vi "Actor Core.vi"(8 "error in":errorcluster, 11 "Tools View in":refnum<class "Tools View.lvclass">) -> (0 "error out":errorcluster, 3 "Actor out":refnum<class "Actor.lvclass">)   [LabVIEW 2020, in "Tools View.lvlib" / "Tools View.lvclass"]
doc: "(<B>Filename</B>: Actor Framework.lvlib:Actor.lvclass:Actor Core.vi)\n\nReceives messages to the actor, reacts to them, and initiates any error handling that may shut the actor down.\n\nDescendant classes may override this VI to append parallel tasks for the actor to complete while it handles messages. Overrides use the Call Parent Method node."
uses:
  Tools View.lvclass
  C:/Program Files/National Instruments/LabVIEW 2020/vi.lib/ActorFramework/Actor/Actor.lvclass
  <vilib>/ActorFramework/Actor/Actor.lvclass
  Tools View.lvclass/Tools View.ctl
  <vilib>/ActorFramework/Actor/Actor.lvclass/Actor.ctl
  <vilib>/ActorFramework/Message Enqueuer/Message Enqueuer.lvclass/Message Enqueuer.ctl
  Type Definitions/Tool Buttons.ctl
  Tools View Messages/Broadcast Tool Buttons Pressed Msg/Broadcast Tool Buttons Pressed Msg.lvclass/Broadcast Tool Buttons Pressed Msg.ctl
  <vilib>/ActorFramework/Message Enqueuer/Init from Existing Queue.vi
  <vilib>/ActorFramework/Message Enqueuer/Enqueue.vi
  Tools View Messages/Broadcast Tool Buttons Pressed Msg/Broadcast Tool Buttons Pressed Msg.lvclass
  C:/Program Files/National Instruments/LabVIEW 2020/vi.lib/ActorFramework/Message/Message.lvclass
  <vilib>/ActorFramework/Message Priority Queue/Priority Enqueue.vi
  <vilib>/ActorFrameworkMVC/Abstract View/Abstract View/Abstract View.lvclass
  <vilib>/ActorFramework/Message Enqueuer/Message Enqueuer.lvclass
panel:
  in  "Disabled Crop Button":bool
  in  "Disabled Deselect Button":bool
  in  "Tool Buttons":T1(radio)
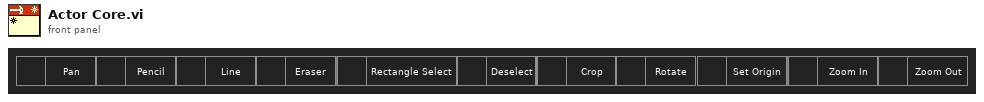
[diagram p1: front panel]
types:
  T1 = enum32{"Pan Button", "Pencil Button", "Line Button", "Eraser Button", "Rectangle Select Button", "Deselect Button", "Crop Button", "Rotate Button", "Set Origin Button", "Zoom In Button", "Zoom Out Button"}
  T2 = enum8{"Enabled", "Disabled", "Disabled and Grayed Out"}
  T3 = typedef "Tool Buttons.ctl" = enum32{"Pan Button", "Pencil Button", "Line Button", "Eraser Button", "Rectangle Select Button", "Deselect Button", "Crop Button", "Rotate Button", "Set Origin Button", "Zoom In Button", "Zoom Out Button"}
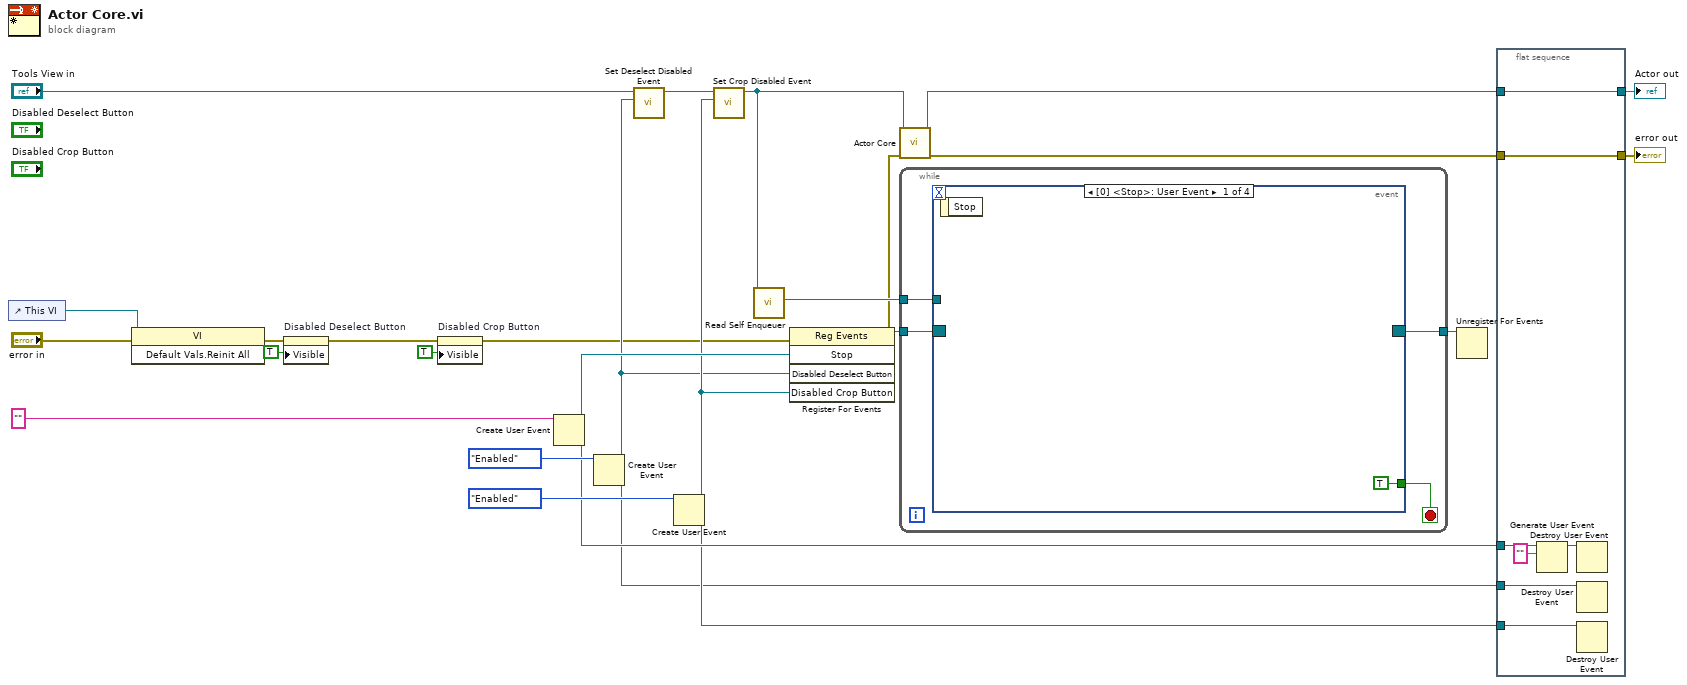
[diagram p0: block diagram]
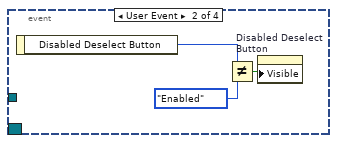
[diagram p2: hidden frame]
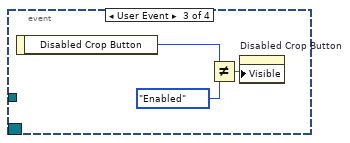
[diagram p3: hidden frame]
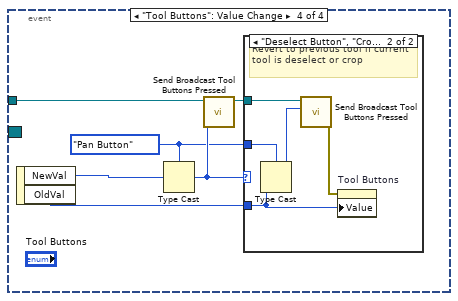
[diagram p4: hidden frame]
diagram:
  n1 = control-ref of="This VI"() -> (w6:refnum<vi>)
  n2 = invoke class="VI" method="Default Vals.Reinit All"(reference=w6, error in="error in") -> (error out=w5:errorcluster)  [unwired: 1 in, 2 out]
  n3 = property on="Disabled Deselect Button" class="Bool"(error in=w5, "Visible"=TRUE) -> (error out=w4:errorcluster)  [unwired: 1 in, 1 out]
  n4 = property on="Disabled Crop Button" class="Bool"(error in=w4, "Visible"=TRUE) -> (error out=w3:errorcluster)  [unwired: 1 in, 1 out]
  n5 = Create User Event(user event datatype="" ("Stop")) -> (user event=w18:refnum<user-event>)  [unwired: 1 in, 1 out]
  n6 = Create User Event(user event datatype=T2."Enabled" ("Disabled Deselect Button")) -> (user event=w9:refnum<user-event>)  [unwired: 1 in, 1 out]
  n7 = call "Set Deselect Disabled Event.vi"("Deselect Disabled Event"=w9, "Tools View in"="Tools View in") -> ("Tools View out"=w11:refnum<class "Tools View.lvclass">)  [unwired: 9 in]
  n8 = Create User Event(user event datatype=T2."Enabled" ("Disabled Crop Button")) -> (user event=w10:refnum<user-event>)  [unwired: 1 in, 1 out]
  n9 = call "Set Crop Disabled Event.vi"("Crop Disabled Event"=w10, "Tools View in"=w11) -> ("Tools View out"=w7:refnum<class "Tools View.lvclass">)  [unwired: 9 in]
  n10 = call <vilib>:"Read Self Enqueuer.vi"("Actor"=w7) -> ("Self Enqueuer"=w19:refnum<class "Message Enqueuer.lvclass">)  [unwired: 10 in]
  n11 = register-events(error in=w3, w18, w9, w10) -> (reference out=w20:refnum<event-registration>, error out=w12:errorcluster)  [unwired: 1 in]
  n12 = call-parent "Actor Core.vi"("error in"=w12, "Abstract View in"=w7) -> ("error out"=w15:errorcluster, "Actor out"=w14:refnum<class "Actor.lvclass">)  [unwired: 8 in]
  n13 = while {
    tunnel: w20 -> [w28]
    tunnel: [w27] -> w21
    tunnel: w19 -> [w25]
    stop <- w26 stop-if-true
    n14 = event shown="[0] <Stop>: User Event" {
      selector: w28 -> [_ _ _ _]
      dyn-events: [_ _ _ _] -> w27
      timeout: _ -> [_ _ _ _]
      tunnel: [TRUE _ _ _] -> w26
      tunnel: w25 -> [_ _ _ w41]
      event User Event {
        n15 = event-data() -> ()  [unwired: 1 in, 1 out]
      }
      event User Event {
        n16 = event-data() -> ("Disabled Deselect Button"=w32:T2)  [unwired: 1 in]
        n17 = Not Equal?(x=w32, y=T2."Enabled") -> (x != y?=w30:bool)
        n18 = property on="Disabled Deselect Button" class="Bool"("Visible"=w30) -> ()  [unwired: 2 in, 2 out]
      }
      event User Event {
        n19 = event-data() -> ("Disabled Crop Button"=w35:T2)  [unwired: 1 in]
        n20 = Not Equal?(x=w35, y=T2."Enabled") -> (x != y?=w33:bool)
        n21 = property on="Disabled Crop Button" class="Bool"("Visible"=w33) -> ()  [unwired: 2 in, 2 out]
      }
      event "Tool Buttons": Value Change {
        w37 = Tool_Buttons."Pan Button" ("Tool Buttons Pressed")
        n22 = event-data() -> ("NewVal"=w40:T1, "OldVal"=w36:T1)  [unwired: 1 in]
        n23 = Type Cast(type=w37, x=w40) -> (*(type *) &x=w39:T3)
        n24 = call "Send Broadcast Tool Buttons Pressed.vi"("Tool Buttons Pressed"=w39, "Message Enqueuer"=w41) -> ("Message Enqueuer out"=w38:refnum<class "Message Enqueuer.lvclass">)  [unwired: 8 in, 1 out]
        n25 = case shown="\"Deselect Button\", \"Crop Button\"" w39 {
          tunnel: w38 -> [_ w44]
          tunnel: w37 -> [_ w45]
          tunnel: w36 -> [_ w43]
          frame Default {
          }
          frame "Deselect Button", "Crop Button" {
            # "Revert to previous tool if current tool is deselect or crop"
            n26 = Type Cast(type=w45, x=w43) -> (*(type *) &x=w46:T3)
            n27 = call "Send Broadcast Tool Buttons Pressed.vi"("Tool Buttons Pressed"=w46, "Message Enqueuer"=w44) -> ("error out"=w42:errorcluster)  [unwired: 8 in, 1 out]
            n28 = property on="Tool Buttons" class="RadioBtnsControl (strict)"(error in=w42, "Value"=w43) -> ()  [unwired: 1 in, 2 out]
          }
        }
      }
    }
  }
  n29 = Unregister For Events(event registration refnum=w21) -> ()  [unwired: 1 in, 1 out]
  n30 = flat-sequence {
    tunnel: w18 -> [w52]
    tunnel: w9 -> [w50]
    tunnel: w10 -> [w49]
    tunnel: w14 -> [w48]
    tunnel: [w48] -> w17
    tunnel: [w47] -> w16
    tunnel: w15 -> [w47]
    frame #0 {
      n31 = Generate User Event(user event=w52, event data cluster="" ("event data")) -> (user event out=w53:refnum<user-event>)  [unwired: 2 in, 1 out]
      n32 = Destroy User Event(user event=w53) -> ()  [unwired: 1 in, 1 out]
      n33 = Destroy User Event(user event=w50) -> ()  [unwired: 1 in, 1 out]
      n34 = Destroy User Event(user event=w49) -> ()  [unwired: 1 in, 1 out]
    }
  }
  "error out" <- w16
  "Actor out" <- w17
